vi "Get pressure.vi"(8 "error in (no error)":errorcluster, 11 "Pressure Control in":refnum<class "Pressure Control.lvclass">) -> (0 "error out":errorcluster, 1 "Uncorrected pressure":dbl, 2 "Pressure":dbl, 3 "Pressure Control out":refnum<class "Pressure Control.lvclass">)   [LabVIEW 2011, in "Pressure Control.lvclass"]
uses:
  Pressure Control.lvclass
  Pressure Control.lvclass/Pressure Control.ctl
  <vilib>/DAQmx/read.llb/DAQmx Read (Analog DBL 1Chan 1Samp).vi
  <vilib>/DAQmx/miscellaneous.llb/DAQmx Fill In Error Info.vi
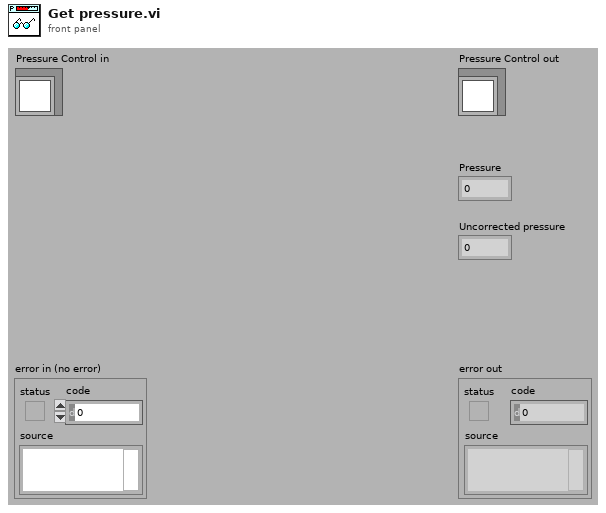
[diagram p1: front panel]
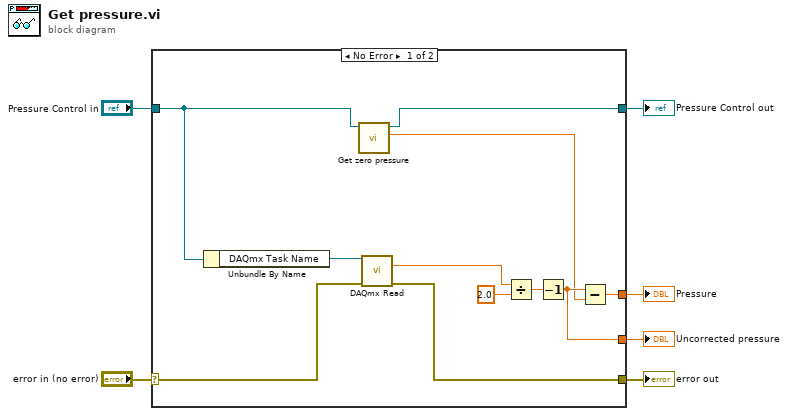
[diagram p0: block diagram]
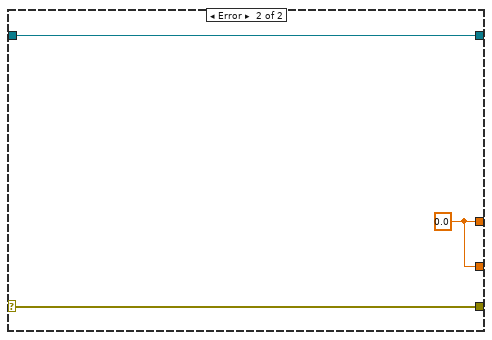
[diagram p2: hidden frame]
diagram:
  n1 = case shown="No Error" "error in (no error)" {
    selector: "error in (no error)" -> [w16 w20]
    tunnel: [w11 w20] -> w5
    tunnel: [w8 w19] -> w3
    tunnel: "Pressure Control in" -> [w9 w19]
    tunnel: [w12 w18] -> w2
    tunnel: [w10 w18] -> w1
    frame No Error {
      n2 = Unbundle By Name(w9) -> ("DAQmx Task Name"=w17:refnum<k21>)
      n3 = call "Get zero pressure.vi"("Pressure Control in"=w9) -> ("Zero pressure level"=w7:dbl, "Pressure Control out"=w8:refnum<class "Pressure Control.lvclass">)  [unwired: 8 in, 1 out]
      n4 = call-poly <vilib>:"DAQmx Read.vi"("task/channels in"=w17, "error in"=w16) -> ("data"=w15:dbl, "error out"=w11:errorcluster)  [unwired: 11 in, 1 out]
      n5 = Divide(x=w15, y=2.0) -> (x/y=w13:dbl)
      n6 = Decrement(x=w13) -> (x-1=w10:dbl)
      n7 = Subtract(x=w10, y=w7) -> (x-y=w12:dbl)
    }
    frame Error {
      w18 = 0.0
    }
  }
  "error out" <- w5
  "Pressure Control out" <- w3
  "Pressure" <- w2
  "Uncorrected pressure" <- w1
